vi "Omron_COMM.vi"(8 "error in":errorcluster, 10 "Write data":string, 11 "COM in":refnum<visa-resource-name>) -> (0 "error out":errorcluster, 2 "Receive data":string, 3 "COM out":refnum<visa-resource-name>)   [LabVIEW 2015]
uses:
  <vilib>/Instr/_visa.llb/VISA Flush IO Buffer Mask.ctl
  Instance           1 18Saved   Omron_COMM .vi
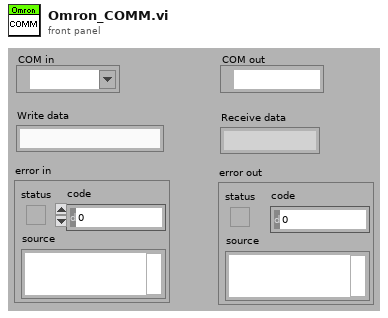
[diagram p1: front panel]
types:
  T1 = typedef "VISA Flush IO Buffer Mask.ctl" = u16
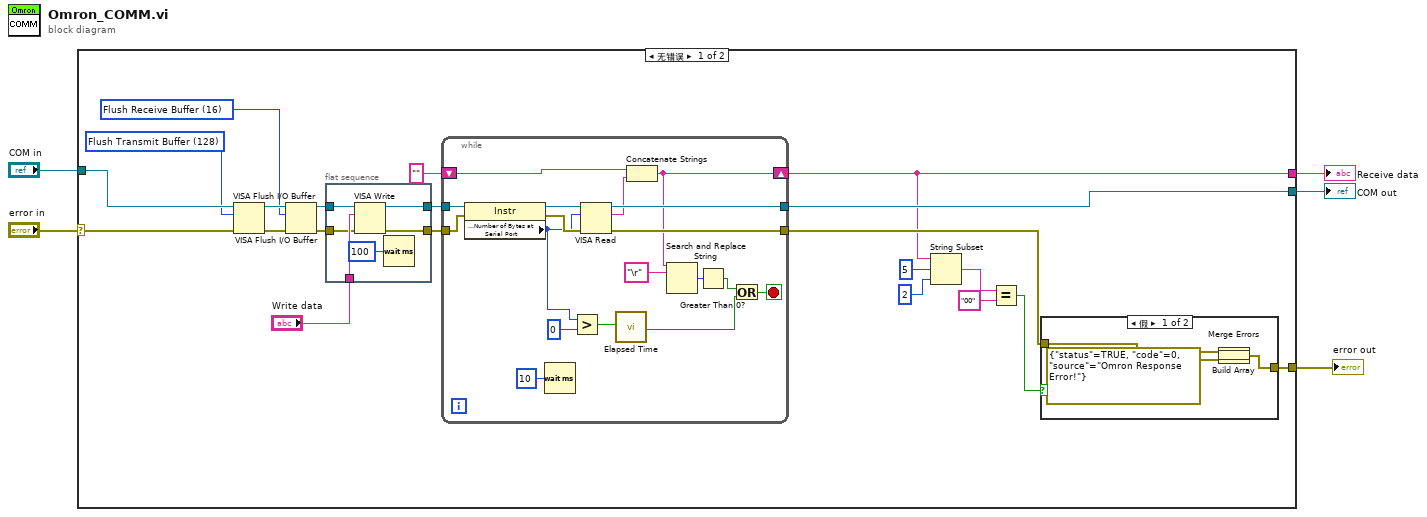
[diagram p0: block diagram]
diagram:
  n1 = case shown="无错误" "error in" {
    selector: "error in" -> [w13 w56]
    tunnel: [w6 _] -> w5
    tunnel: [w26 w56] -> w4
    tunnel: [w8 w57] -> w3
    tunnel: "COM in" -> [w20 w57]
    frame No Error {
      w9 = T1 16 items=["Flush Receive Buffer"=16, "Write Transmit Buffer to Device"=32, "Flush Receive Buffer (No I/O)"=64, "Flush Transmit Buffer"=128] ("Mask")
      w14 = T1 128 items=["Flush Receive Buffer"=16, "Write Transmit Buffer to Device"=32, "Flush Receive Buffer (No I/O)"=64, "Flush Transmit Buffer"=128] ("Mask")
      n2 = VISA Flush I/O Buffer(VISA resource name=w20, mask (16)=w14, error in (no error)=w13) -> (VISA resource name out=w15:refnum<visa-resource-name>, error out=w11:errorcluster)
      n3 = VISA Flush I/O Buffer(VISA resource name=w15, mask (16)=w9, error in (no error)=w11) -> (VISA resource name out=w12:refnum<visa-resource-name>, error out=w10:errorcluster)
      n4 = flat-sequence {
        tunnel: [w32] -> w19
        tunnel: [w31] -> w18
        tunnel: "Write data" -> [w30]
        tunnel: w12 -> [w29]
        tunnel: w10 -> [w28]
        frame #0 {
          n5 = VISA Write(VISA resource name=w29, write buffer=w30, error in (no error)=w28) -> (VISA resource name out=w31:refnum<visa-resource-name>, error out=w32:errorcluster)  [unwired: 1 out]
          n6 = Wait (ms)(milliseconds to wait=u32 100) -> ()  [unwired: 1 out]
        }
      }
      n7 = while {
        tunnel: [w51] -> w8
        tunnel: [w50] -> w7
        tunnel: w18 -> [w55]
        tunnel: w19 -> [w54]
        shift-right: [w42] -> w6
        shift-left: "" -> [w49]
        stop <- w45 stop-if-true
        n8 = property class="Instr"(reference=w55, error in=w54) -> (reference out=w53:refnum<visa-resource-name>, error out=w52:errorcluster, "Serial Settings:Number of Bytes at Serial Port"=w38:u32)
        n9 = Wait (ms)(milliseconds to wait=u32 10) -> ()  [unwired: 1 out]
        n10 = Greater?(x=w38, y=u32 0) -> (0:w40:bool)
        n11 = VISA Read(VISA resource name=w53, byte count=w38, error in (no error)=w52) -> (VISA resource name out=w51:refnum<visa-resource-name>, read buffer=w48:string, error out=w50:errorcluster)  [unwired: 1 out]
        n12 = call "Elapsed Time"("Reset"=w40) -> ("Time has Elapsed"=w43:bool)  [unwired: 11 in, 7 out]
        n13 = Concatenate Strings(w49, w48) -> (w42:string)
        n14 = Search and Replace String(input string=w42, search string="\r") -> (number of replacements=w46:i32)  [unwired: 6 in, 3 out]
        n15 = Greater Than 0?(x=w46) -> (x > 0?=w41:bool)
        n16 = Or(x=w41, y=w43) -> (x .or. y?=w45:bool)
      }
      n17 = String Subset(string=w6, offset (0)=5, length (rest)=2 ("length (rest)")) -> (substring=w23:string)
      n18 = Equal?(x=w23, y="00") -> (x = y?=w25:bool)
      n19 = case shown="假" w25 {
        tunnel: w7 -> [w36 w37]
        tunnel: [w34 w37] -> w26
        frame False {
          n20 = Build Array(w36, errorcluster {"status"=TRUE, "code"=0, "source"="Omron Response Error!"} ("error out")) -> (w33:errorcluster[])
          n21 = Merge Errors(w33) -> (w34:errorcluster)
        }
        frame True {
        }
      }
    }
    frame Error {
    }
  }
  "Receive data" <- w5
  "error out" <- w4
  "COM out" <- w3
